vi "Generate Output and Read.vi"() -> ()   [LabVIEW 2020]
uses:
  <userlib>/DAQNavi Polymorphic VI/create/DAQNavi Create Channel(AO-Voltage).vi
  <userlib>/DAQNavi Polymorphic VI/create/DAQNavi Create Channel(AI-Voltage).vi
  <userlib>/DAQNavi Polymorphic VI/write/DAQNavi Write (Analog DBL 1Chan 1Samp).vi
  <userlib>/DAQNavi Polymorphic VI/read/DAQNavi Read (Analog Wfm 1Chan 1Samp).vi
panel:
  in  "Command":dbl(slide)=5.0 scale=0.0..10.0
  out "value range Input":string="+/- 10 V" caption="property value"
  out "physical channels Input":string="DemoDevice,BID#0/ai0:0" caption="property value"
  in  "stop":bool
  out "Waveform Chart":waveform(dbl)(graph)
  out "error out":errorcluster
  out "value range Output":string="+/- 5 V" caption="property value"
  out "physical channels Output":string="DemoDevice, BID#0/ao1:1" caption="property value"
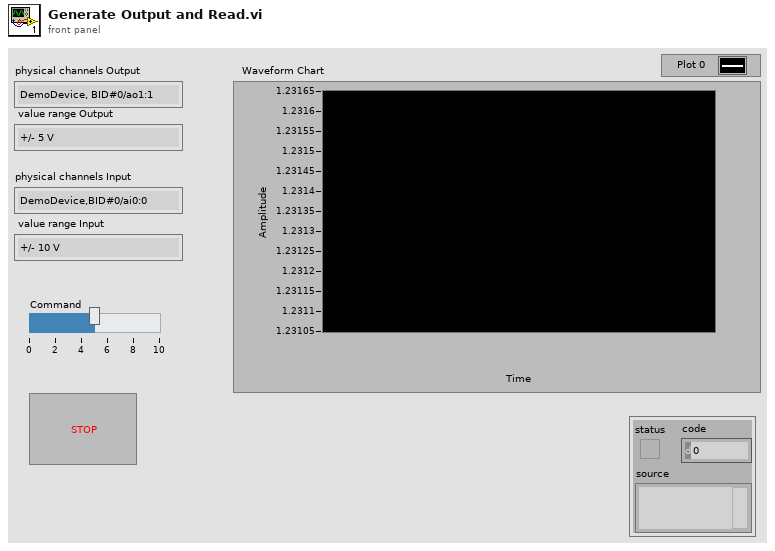
[diagram p1: front panel]
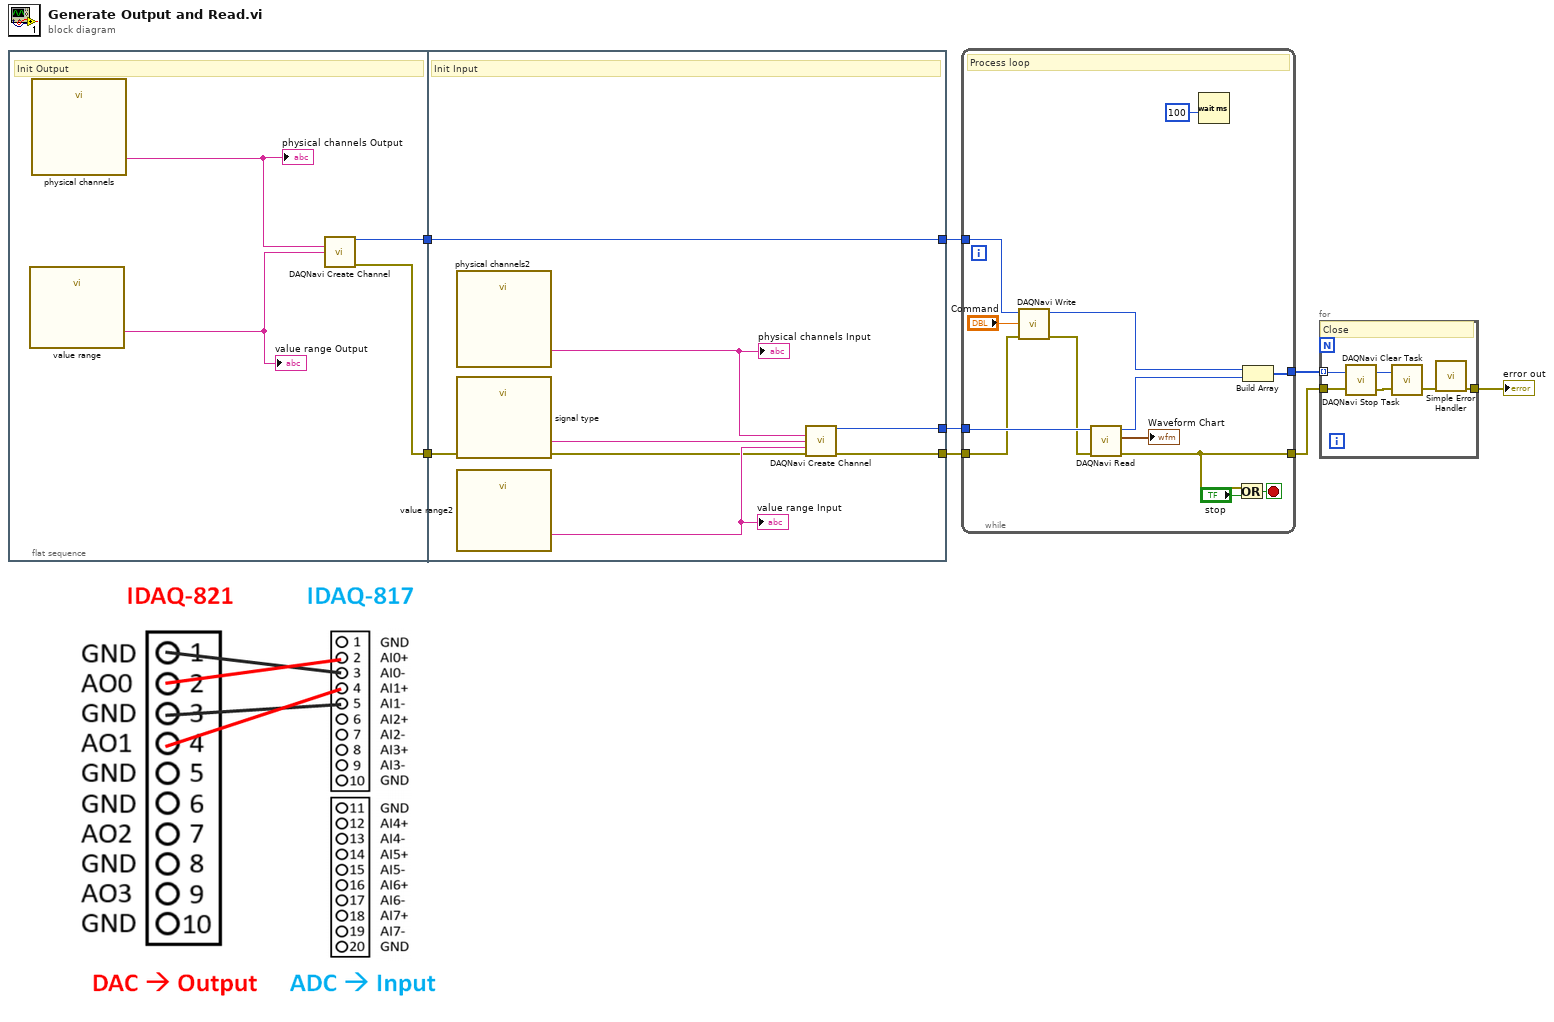
[diagram p0: block diagram]
diagram:
  n1 = flat-sequence {
    tunnel: [w12] -> w8
    tunnel: [w11] -> w7
    tunnel: [w19] -> w4
    tunnel: w8 -> [w19]
    tunnel: w7 -> [w15]
    tunnel: [w14] -> w5
    tunnel: [w13] -> w6
    frame #0 {
      # "Init Output"
      n2 = call "value range"() -> ("property value"=w10:string)  [unwired: 1 out]
      "value range Output" <- w10
      n3 = call "physical channels"() -> ("property value"=w9:string)  [unwired: 1 out]
      "physical channels Output" <- w9
      n4 = call-poly <userlib>:"DAQNavi Create Channel.vi"("physical channels"=w9, "value range"=w10) -> ("task out"=w12:i32, "error out"=w11:errorcluster)  [unwired: 3 in, 9 out]
    }
    frame #1 {
      # "Init Input"
      n5 = call "physical channels2"() -> ("property value"=w16:string)  [unwired: 1 out]
      "physical channels Input" <- w16
      n6 = call "signal type"() -> ("property value"=w18:string)  [unwired: 1 out]
      n7 = call "value range2"() -> ("property value"=w17:string)  [unwired: 1 out]
      "value range Input" <- w17
      n8 = call-poly <userlib>:"DAQNavi Create Channel.vi"("physical channels"=w16, "signal type"=w18, "value range"=w17, "error in (no error)"=w15) -> ("task out"=w14:i32, "error out"=w13:errorcluster)  [unwired: 1 in, 9 out]
    }
  }
  n9 = while {
    tunnel: w5 -> [w32]
    tunnel: w6 -> [w25]
    tunnel: w4 -> [w26]
    tunnel: [w21] -> w1
    tunnel: [w20] -> w3
    stop <- w31 stop-if-true
    # "Process loop"
    n10 = call-poly <userlib>:"DAQNavi Write.vi"("error in (no error)"=w25, "data"="Command", "task in"=w26) -> ("error out"=w24:errorcluster, "task out"=w23:i32)  [unwired: 1 in, 6 out]
    n11 = call-poly <userlib>:"DAQNavi Read.vi"("error in (no error)"=w24, "task in"=w32) -> ("error out"=w21:errorcluster, "data"=→"Waveform Chart":waveform(dbl), "task out"=w22:i32)  [unwired: 2 in, 5 out]
    n12 = Wait (ms)(milliseconds to wait=u32 100) -> ()  [unwired: 1 out]
    n13 = Or(x=w21, y="stop") -> (x .or. y?=w31:bool)
    n14 = Build Array(w23, w22) -> (w20:i32[])
  }
  n15 = for {
    tunnel: w3 -> [w36] mode=indexing
    tunnel: [w35] -> w2
    tunnel: w1 -> [w34]
    # "Close"
    n16 = call <userlib>:"DAQNavi Stop Task.vi"("error in (no error)"=w34, "task in"=w36) -> ("error out"=w38:errorcluster, "task out"=w33:i32)
    n17 = call <userlib>:"DAQNavi Clear Task.vi"("error in (no error)"=w38, "task in"=w33) -> ("error out"=w37:errorcluster)  [unwired: 1 out]
    n18 = call <vilib>:"Simple Error Handler.vi"("error in (no error)"=w37) -> ("error out"=w35:errorcluster)  [unwired: 2 in, 6 out]
  }
  "error out" <- w2
